vi "Launch Nested Model.vi"(6 "Confirm Shutdown? (T)":bool=TRUE, 8 "error in (no error)":errorcluster, 9 "Auto-stop? (T)":bool=TRUE, 10 "Model to Launch":refnum<class "IModel.lvclass">, 11 "IModel in":refnum<class "IModel.lvclass">) -> (0 "error out":errorcluster, 2 "Nested Model Enqueuer":refnum<class "Message Enqueuer.lvclass">, 3 "IModel out":refnum<class "IModel.lvclass">)   [LabVIEW 2019, in "IModel.lvlib" / "IModel.lvclass"]
uses:
  <vilib>/gpm_packages/@cs/mva-core/Source/IModel/IModel/IModel.lvclass
  C:/Program Files/National Instruments/LabVIEW 2019/vi.lib/ActorFramework/Actor/Actor.lvclass
  C:/Program Files/National Instruments/LabVIEW 2019/vi.lib/gpm_packages/@cs/mva-core/Source/IObserver/IObserver/IObserver.lvclass
  <vilib>/ActorFramework/Message Enqueuer/Message Enqueuer.lvclass
  <vilib>/gpm_packages/@cs/mva-core/Source/IModel/IModel/IModel.lvclass/IModel.ctl
  <vilib>/gpm_packages/@cs/mva-core/Source/IObserver/IObserver/IObserver.lvclass/IObserver.ctl
  <vilib>/gpm_packages/@cs/event-logger/Source/Composed Log/LoggerReference/LoggerReference.lvclass/LoggerReference.ctl
  <vilib>/gpm_packages/@cs/mva-core/Source/IObserver/IObserver/Transfer Observer Resources.vi
  <vilib>/gpm_packages/@cs/event-logger/Source/Composed Log/LoggerReference/Log Event.vi
  <vilib>/gpm_packages/@cs/event-logger/Source/Composed Log/LoggerReference/Log.vi
  <vilib>/gpm_packages/@cs/event-logger/Source/Composed Log/LoggerReference/Get Valid Event Time.vi
  <vilib>/gpm_packages/@cs/event-logger/Source/Composed Log/LoggerReference/Remove Stale Logs.vi
  <vilib>/ActorFramework/Actor/Actor.lvclass
  <vilib>/gpm_packages/@cs/mva-core/Source/IObserver/IObserver/IObserver.lvclass
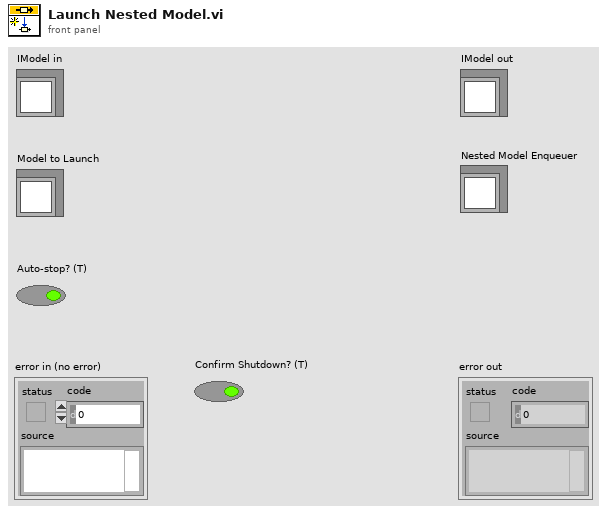
[diagram p1: front panel]
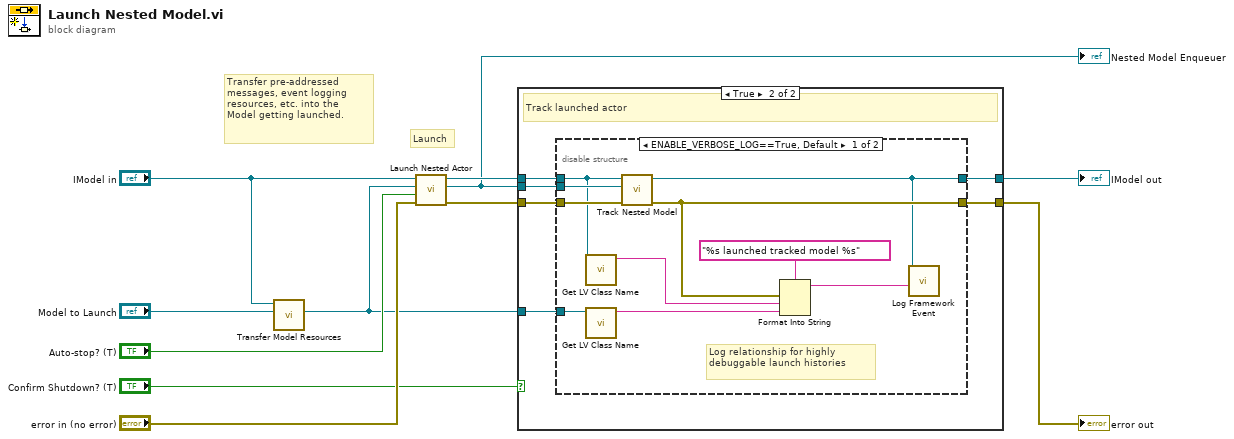
[diagram p0: block diagram]
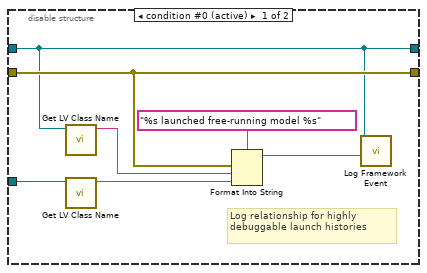
[diagram p3: hidden frame]
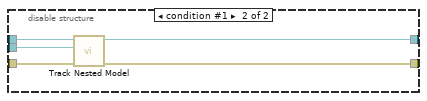
[diagram p4: hidden frame]
diagram:
  # "Launch"
  # "Transfer pre-addressed\nmessages, event logging\nresources, etc. into the\nModel getting launched."
  n1 = call <vilib>:"Transfer Model Resources.vi"("Recipient Model In"="Model to Launch", "Running Model"="IModel in") -> ("Recipient Model Out"=w1:refnum<class "IModel.lvclass">)  [unwired: 9 in]
  n2 = call <vilib>:"Launch Nested Actor.vi"("error in (no error)"="error in (no error)", "Auto-stop? (T)"="Auto-stop? (T)", "Nested Actor"=w1, "Caller Actor in"="IModel in") -> ("error out"=w4:errorcluster, "Nested Actor's Enqueuer"=w7:refnum<class "Message Enqueuer.lvclass">, "Caller Actor out"=w9:refnum<class "IModel.lvclass">)  [unwired: 5 in]
  "Nested Model Enqueuer" <- w7
  n3 = case shown="True" "Confirm Shutdown? (T)" {
    tunnel: w9 -> [w16 w30]
    tunnel: [w14 w29] -> w8
    tunnel: w7 -> [_ w26]
    tunnel: w4 -> [w15 w27]
    tunnel: [w13 w28] -> w3
    tunnel: w1 -> [w12 w31]
    frame False {
      # "Do not track"
      n4 = disable-structure shown="REMOVE_FRAMEWORK_LOG==True" {
        disable-tunnel: w12 -> [w23 _]
        disable-tunnel: w16 -> [w17 w25]
        disable-tunnel: [w17 w25] -> w14
        disable-tunnel: [w18 w24] -> w13
        disable-tunnel: w15 -> [w18 w24]
        frame condition #0 (active) {
          # "Log relationship for highly\ndebuggable launch histories"
          n5 = call <vilib>:"Get LV Class Name.vi"("object"=w17) -> ("class name"=w22:string)  [unwired: 9 in, 1 out]
          n6 = call <vilib>:"Get LV Class Name.vi"("object"=w23) -> ("class name"=w21:string)  [unwired: 9 in, 1 out]
          n7 = Format Into String(format string="%s launched free-running model %s", error in=w18, w22, w21) -> (resulting string=w19:string)  [unwired: 1 in, 1 out]
          n8 = call <vilib>:"Log Framework Event.vi"("Data To Log"=w19, "IObserver in"=w17) -> ()  [unwired: 9 in, 1 out]
        }
        frame condition #1 {
        }
      }
    }
    frame True {
      # "Track launched actor"
      n9 = disable-structure shown="ENABLE_VERBOSE_LOG==True, Default" {
        disable-tunnel: w31 -> [w41 _]
        disable-tunnel: w30 -> [w32 w46]
        disable-tunnel: [w33 w43] -> w29
        disable-tunnel: [w36 w42] -> w28
        disable-tunnel: w27 -> [w35 w45]
        disable-tunnel: w26 -> [w34 w44]
        frame condition #0 (active) {
          # "Log relationship for highly\ndebuggable launch histories"
          n10 = call <vilib>:"Get LV Class Name.vi"("object"=w32) -> ("class name"=w40:string)  [unwired: 9 in, 1 out]
          n11 = call <vilib>:"Get LV Class Name.vi"("object"=w41) -> ("class name"=w39:string)  [unwired: 9 in, 1 out]
          n12 = call <vilib>:"Track Nested Model.vi"("error in (no error)"=w35, "Nested Model Enqueuer"=w34, "IModel in"=w32) -> ("error out"=w36:errorcluster, "IModel out"=w33:refnum<class "IModel.lvclass">)  [unwired: 7 in]
          n13 = Format Into String(format string="%s launched tracked model %s", error in=w36, w40, w39) -> (resulting string=w37:string)  [unwired: 1 in, 1 out]
          n14 = call <vilib>:"Log Framework Event.vi"("Data To Log"=w37, "IObserver in"=w33) -> ()  [unwired: 9 in, 1 out]
        }
        frame condition #1 {
          n15 = call <vilib>:"Track Nested Model.vi"("error in (no error)"=w45, "Nested Model Enqueuer"=w44, "IModel in"=w46) -> ("error out"=w42:errorcluster, "IModel out"=w43:refnum<class "IModel.lvclass">)  [unwired: 7 in]
        }
      }
    }
  }
  "error out" <- w3
  "IModel out" <- w8
